vi "Set OutputPLC.vi"(0 "Address In":i32=20, 1 "Array 2":T1=[enum."電流量測完成產品OK_21", enum."S2站Format 執行_23", enum."S2 Format OK_24"], 2 "Sat Coils":bool[](array[boolean])=[TRUE], 3 "error in (no error)":errorcluster) -> (10 "Error Out":errorcluster[](array[cluster]))   [LabVIEW 2019, in "LineScan.lvclass"]
uses:
  FlowCtrl Class/LineScan/LineScan.lvclass
  Ctrl/Output to PLC.ctl
  Ctrl/S2 Station IO.ctl
  Ctrl/ModbusCmd.ctl
panel:
  in  "Set Out":enum16{""}[](array[ring])
  in  "Array 3":T1=[enum."電流量測完成產品OK_21", enum."S2站Format 執行_23", enum."S2 Format OK_24"]
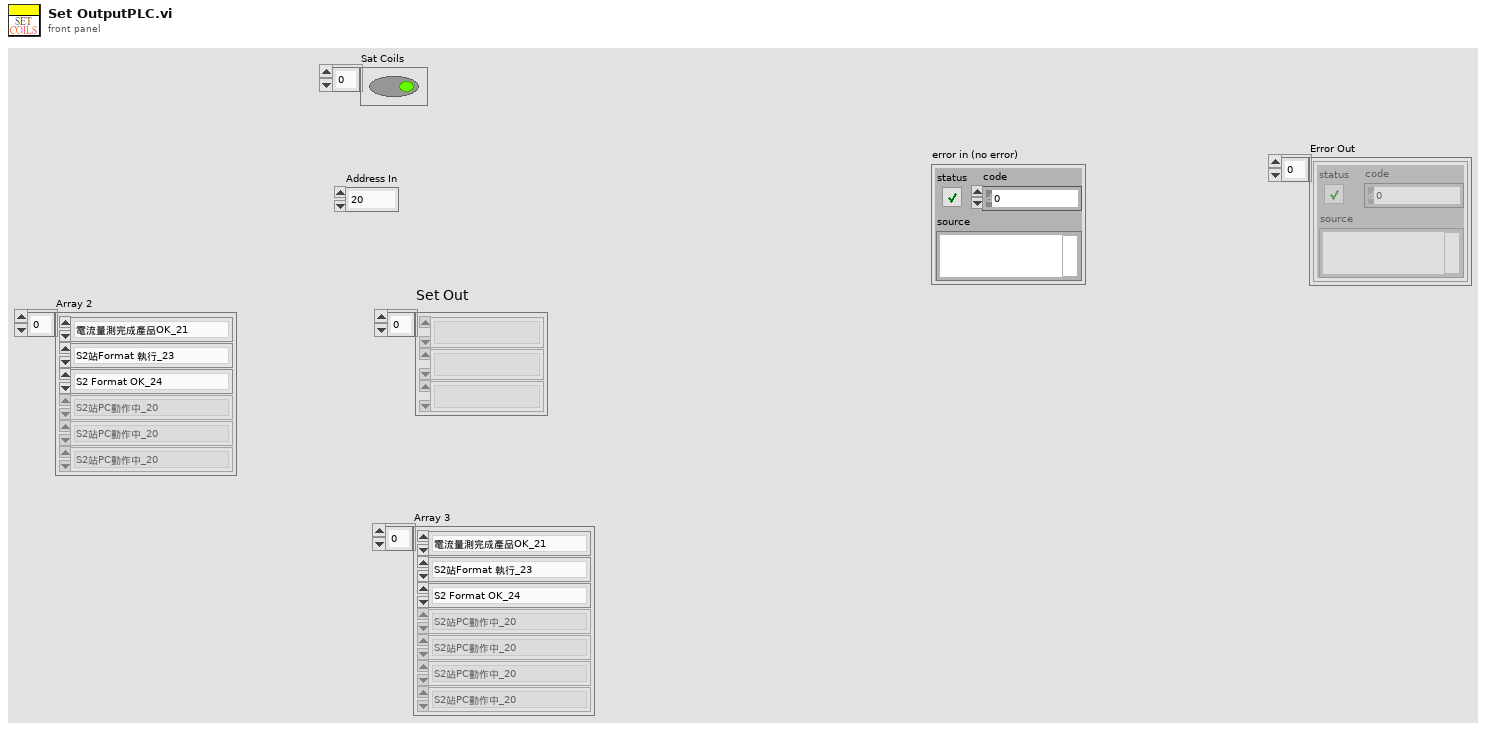
[diagram p1: front panel]
types:
  T1 = typedef "Output to PLC.ctl" = T2[]
  T2 = typedef "S2 Station IO.ctl" = enum16{"S2站PC動作中_20", "電流量測完成產品OK_21", "電流量測完成產品NG_22", "S2站Format 執行_23", "S2 Format OK_24", "S2 Format NG_25", "S2站燒入執行_26", "S2站燒入OK_27", "S2站燒入NG_28", "S2站動作完成_29", "S3 PC動作中_30", "S3 Format 此站執行_31", "S3 Format OK_32", "S3 Format NG_33", "S3 燒入程式 此站執行_34", "S3 燒入程式 OK_35", "S3 燒入程式 NG_36", "S3 備用_37", "S3 備用_38", "S3 動作完成_39", "S4 PC動作中_40", "S4 量測完成 產品正常_41", "S4 量測完成 產品NG_42", "S4 Format 此站執行_43", "S4 Format OK_44", "S4 Format NG_45", "S4 燒入 此站不執行_46", "S4 燒入程式 OK_47", "S4 燒入程式 NG_48", "S4 藍芽Scan OK_49", "S4 藍芽Scan NG_50", "S4 動作完成_51", "給PLC要量電流訊號", "給PLC要量電壓訊號"}
  T3 = cluster{"starting address":u16, "number of inputs":u16, "Sat Coils":bool[], "Holding Registers":u16[]}
  T4 = typedef "ModbusCmd.ctl" = enum16{"Connect", "Disconnect", "Init", "Fetch Basic Objects", "Fetch Input Refisters", "Fetch Discrete Inputs", "Set Coils", "Set Holding Registers", "Write Single Holding", "Exit"}
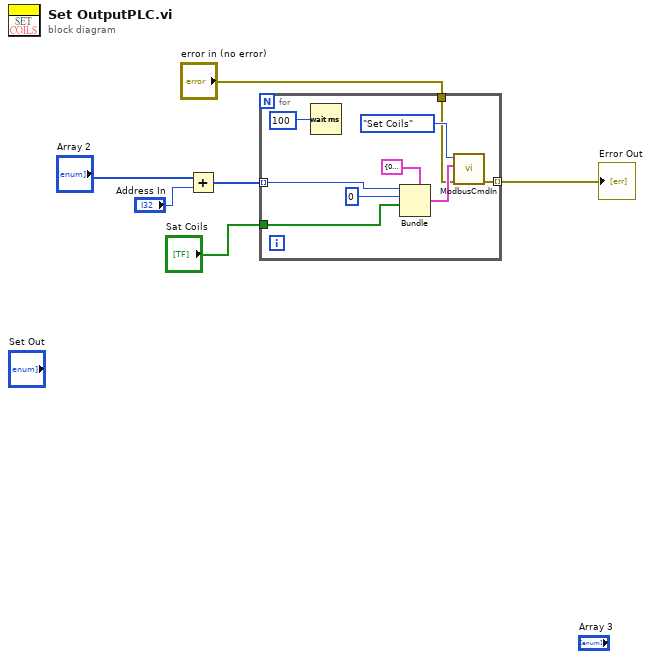
[diagram p0: block diagram]
diagram:
  n1 = Add(x="Array 2", y="Address In") -> (x+y=w5:i32[])
  n2 = for {
    tunnel: [w10] -> w4 mode=indexing
    tunnel: w5 -> [w9] mode=indexing
    tunnel: "Sat Coils" -> [w8]
    tunnel: "error in (no error)" -> [w7]
    n3 = Wait (ms)(milliseconds to wait=100) -> ()  [unwired: 1 out]
    n4 = Bundle(cluster=T3 {"starting address"=0, "number of inputs"=0, "Sat Coils"=[], "Holding Registers"=[]} ("data"), "starting address"=w9, "number of inputs"=u16 0, "Sat Coils"=w8) -> (w13:T3)  [unwired: 1 in]
    n5 = call "ModbusCmdIn.vi"("error in (no error)"=w7, "data"=w13, "Enum"=ModbusCmd."Set Coils") -> ("error out"=w10:errorcluster)  [unwired: 8 in]
  }
  "Error Out" <- w4
